vi "Open.vi"(8 "ErrorIn":errorcluster caption="Error In(no Error)", 10 "Path":path caption="Attribute1", 11 "ReferenceIn":refnum<class "ErrorDefinitionSQLite.lvclass"> caption="Reference In") -> (0 "ErrorOut":errorcluster caption="Error Out", 3 "ReferenceOut":refnum<class "ErrorDefinitionSQLite.lvclass"> caption="Reference Out")   [LabVIEW 2018, in "ErrorDefinitionSQLite.lvclass"]
uses:
  ErrorDefinitionSQLite.lvclass
  <vilib>/drjdpowell/SQLite Library/SQL Connection/Open (path).vi
  <vilib>/drjdpowell/SQLite Library/SQL Connection/Open (string).vi
  <vilib>/AdvancedString/Path To Command Line String.vi
  <vilib>/drjdpowell/SQLite Library/SQL Connection/Execute SQL (No results).vi
  <vilib>/drjdpowell/SQLite Library/SQL Connection/Connection.lvclass
  <vilib>/drjdpowell/SQLite Library/SQLite.lvlib
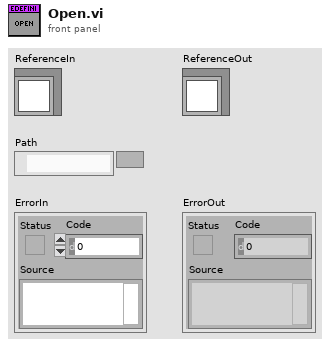
[diagram p1: front panel]
types:
  T1 = enum16{"New or existing", "Existing", "Read only"}
  T2 = typedef "ErrorDefinitionSQLite.lvclass/ObjectAttributes.ctl" = cluster{"Path":path, "SQLiteRef":refnum<class "Connection.lvclass">, "EndOfRange":i32, "DefaultLibrarySize":i32, "StartOfRange":i32}
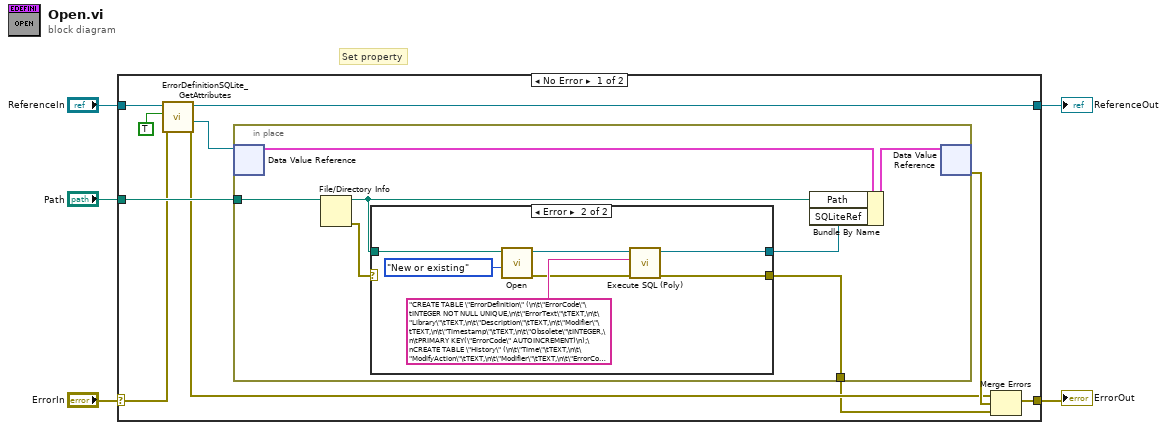
[diagram p0: block diagram]
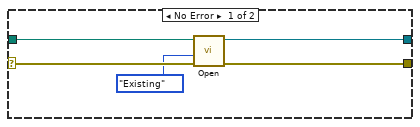
[diagram p2: hidden frame]
diagram:
  # "Set property"
  n1 = case shown="No Error" "ErrorIn" {
    selector: "ErrorIn" -> [w9 w36]
    tunnel: [w13 w36] -> w4
    tunnel: [w11 w35] -> w2
    tunnel: "ReferenceIn" -> [w12 w35]
    tunnel: "Path" -> [w15 _]
    frame No Error {
      n2 = call "ErrorDefinitionSQLite_GetAttributes.vi"("ErrorIn"=w9, "OnlyGetDVRReference"=TRUE ("OnlyGetDvrReference(False)"), "Reference in"=w12) -> ("ErrorOut"=w8:errorcluster, "DataRef"=w10:refnum<data-value>, "Reference out"=w11:refnum<class "ErrorDefinitionSQLite.lvclass">)  [unwired: 5 in, 1 out]
      n3 = in-place {
        in-place-border: w15 -> [w20]
        in-place-border: [w17] -> w6
        n4 = in-place-dvr #1(w10) -> (w22:T2)  [unwired: 1 out]
        n5 = File/Directory Info(path=w20) -> (path out=w18:path, error out=w19:errorcluster)  [unwired: 1 in, 5 out]
        n6 = case shown="Error" w19 {
          selector: w19 -> [w27 _]
          tunnel: w18 -> [w25 w34]
          tunnel: [w26 w29] -> w17
          tunnel: [w24 w28] -> w16
          frame No Error {
            n7 = call-poly <vilib>:"Open.vi"("error in (no error)"=w27, "File Option"=T1."Existing", "db file"=w25) -> ("error out"=w26:errorcluster, "SQLite Connection"=w24:refnum<class "Connection.lvclass">)  [unwired: 7 in]
          }
          frame Error {
            n8 = call-poly <vilib>:"Open.vi"("File Option"=T1."New or existing", "db file"=w34) -> ("error out"=w30:errorcluster, "SQLite Connection"=w32:refnum<class "Connection.lvclass">)  [unwired: 8 in]
            n9 = call-poly <vilib>:"Execute SQL (Poly).vi"("error in (no error)"=w30, "SQL"="CREATE TABLE \"ErrorDefinition\" (\n\t\"ErrorCode\"\tINTEGER NOT NULL UNIQUE,\n\t\"ErrorText\"\tTEXT,\n\t\"Library\"\tTEXT,\n\t\"Description\"\tTEXT,\n\t\"Modifier\"\tTEXT,\n\t\"Timestamp\"\tTEXT,\n\t\"Obsolete\"\tINTEGER,\n\tPRIMARY KEY(\"ErrorCode\" AUTOINCREMENT)\n);\nCREATE TABLE \"History\" (\n\t\"Time\"\tTEXT,\n\t\"ModifyAction\"\tTEXT,\n\t\"Modifier\"\tTEXT,\n\t\"ErrorCode\"\tINTEGER,\n\t\"ErrorText\"\tTEXT,\n\t\"Library\"\tTEXT,\n\t\"Description\"\tTEXT\n, \"LibraryPK\"\tINTEGER);\nCREATE TABLE \"LibraryRanges\" (\n\t\"PK\"\tINTEGER,\n\t\"LibraryName\"\tTEXT,\n\t\"StartRange\"\tINTEGER,\n\t\"EndRange\"\tINTEGER,\n\t\"Obsolete\"\tINTEGER,\n\t\"Full\"\tINTEGER,\n\t\"Timestamp\"\tTEXT,\n\t\"Modifier\"\tTEXT,\n\tPRIMARY KEY(\"PK\")\n)", "SQLite Connection in"=w32) -> ("error out"=w29:errorcluster, "SQLite Connection"=w28:refnum<class "Connection.lvclass">)  [unwired: 7 in]
          }
        }
        n10 = Bundle By Name(cluster=w22, "Path"=w18, "SQLiteRef"=w16) -> (w21:T2)
        n11 = in-place-dvr #1(w21) -> (w14:errorcluster)  [unwired: 1 out]
      }
      n12 = Merge Errors(w8, w14, w6) -> (w13:errorcluster)
    }
    frame Error {
    }
  }
  "ErrorOut" <- w4
  "ReferenceOut" <- w2
